vi "Frame Load Bmp and Img.vi"(8 "error in (no error)":errorcluster, 9 "PNG Path":path, 10 "File String":string, 11 "LF2R IDE in":refnum<class "Main Panel.lvclass">) -> (0 "error out":errorcluster, 3 "LF2R IDE out":refnum<class "Main Panel.lvclass">)   [LabVIEW 2018, in "Main Panel.lvlib" / "Main Panel.lvclass"]
uses:
  Main Panel.lvclass
  <vilib>/picture/picture.llb/imagedata.ctl
  Main Panel.lvclass/Main Panel.ctl
  Frame Analizer/Data Parser.lvclass
  Picture Process/Picture Process.lvclass
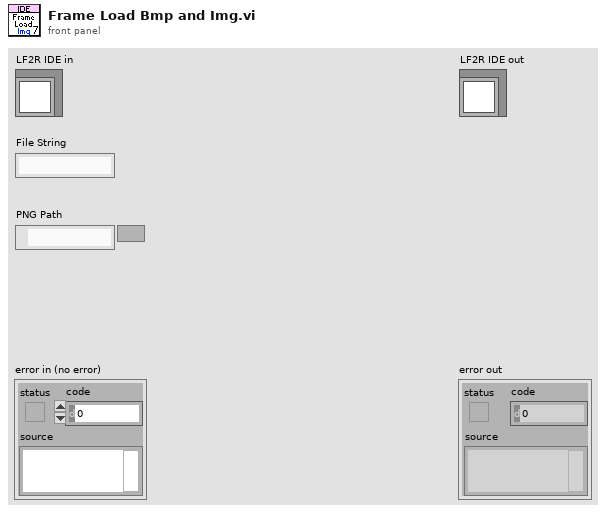
[diagram p1: front panel]
types:
  T1 = typedef "imagedata.ctl" = cluster{"image type":i32, "image depth":i32, "image":u8[], "mask":u8[], "colors":u32[], "Rectangle":cluster{"left":i16, "top":i16, "right":i16, "bottom":i16}}
  T2 = typedef "Data Parser.lvclass/Bmp data.ctl" = cluster{"File Data":T3[], "resized":string, "default_centerx":string, "default_centery":string}
  T3 = typedef "Data Parser.lvclass/Bmp File Data.ctl" = cluster{"Pic Start":i32, "Pic End":i32, "Json Path":string, "w":i32, "h":i32, "row":i32, "col":i32}
  T4 = typedef "Image Json Parser.lvclass/Img Json Data.ctl" = cluster{"frames":T5[], "meta":T6}
  T5 = typedef "Image Json Parser.lvclass/Img Json Frames.ctl" = cluster{"frame":cluster{"x":i32, "y":i32, "w":i32, "h":i32}, "rotated":bool, "trimmed":bool, "spriteSourceSize":cluster{"x":i32, "y":i32, "w":i32, "h":i32}, "sourceSize":cluster{"w":i32, "h":i32}}
  T6 = typedef "Image Json Parser.lvclass/Img Json Meta.ctl" = cluster{"app":string, "version":string, "image":string, "format":string, "size":cluster{"w":i32, "h":i32}, "scale":string}
  T7 = cluster{"image data":T1, "24-bit pixmap":u32[][]}
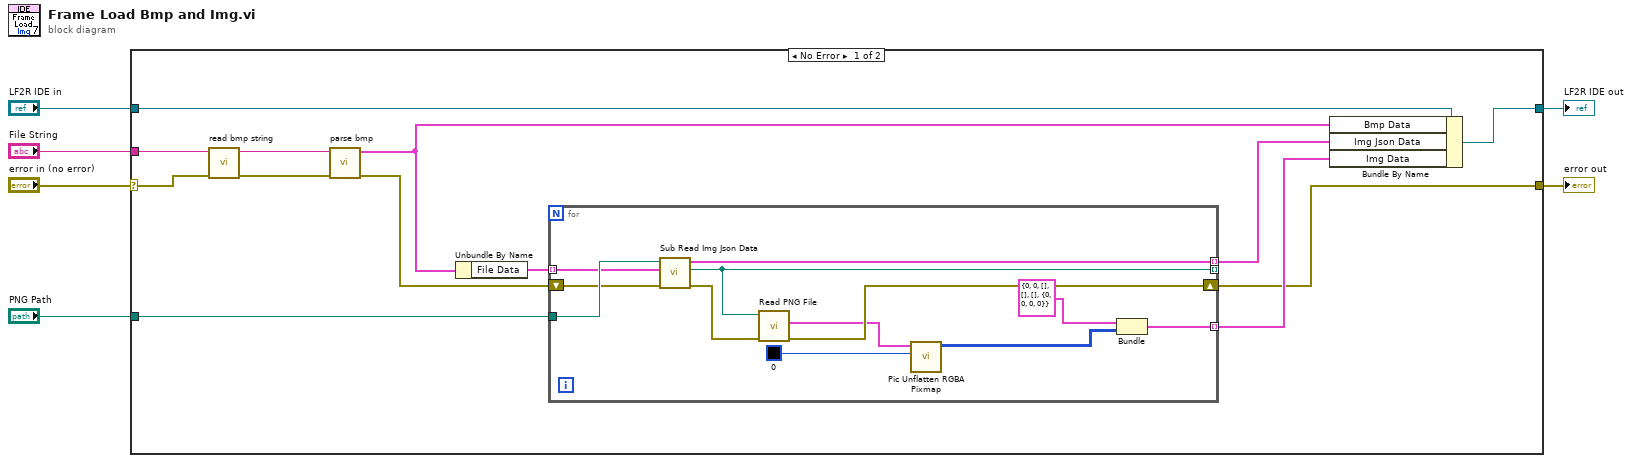
[diagram p0: block diagram]
diagram:
  n1 = case shown="No Error" "error in (no error)" {
    selector: "error in (no error)" -> [w15 w33]
    tunnel: [w7 w33] -> w5
    tunnel: [w14 w32] -> w3
    tunnel: "LF2R IDE in" -> [w19 w32]
    tunnel: "File String" -> [w16 _]
    tunnel: "PNG Path" -> [w13 _]
    frame No Error {
      n2 = call "read bmp string.vi"("error in"=w15, "file string"=w16) -> ("error out"=w17:errorcluster, "<bmp> string"=w18:string)  [unwired: 7 in, 1 out]
      n3 = call "parse bmp.vi"("error in (no error)"=w17, "<bmp> string"=w18) -> ("error out"=w9:errorcluster, "bmp data"=w12:T2)  [unwired: 8 in]
      n4 = Unbundle By Name(w12) -> ("File Data"=w11:T3[])
      n5 = for {
        tunnel: w13 -> [w31]
        tunnel: [w28] -> w10 mode=indexing
        shift-right: [w22] -> w7
        shift-left: w9 -> [w30]
        tunnel: w11 -> [w29] mode=indexing
        tunnel: [w27] -> _ mode=indexing
        tunnel: [w25] -> w8 mode=indexing
        n6 = call "Sub Read Img Json Data.vi"("error in"=w30, "File Data"=w29, "PNG Path"=w31) -> ("error out"=w26:errorcluster, "Image Path"=w27:path, "Json Data"=w28:T4)  [unwired: 6 in]
        n7 = call <vilib>:"Read PNG File.vi"("error in (no error)"=w26, "path to PNG file"=w27) -> ("error out"=w22:errorcluster, "image data"=w21:T1)  [unwired: 7 in, 1 out]
        n8 = call "Pic Unflatten RGBA Pixmap.vi"("BG Color"=u32 0, "32-bit image data (ARGB)"=w21) -> ("24-bit pixmap"=w24:u32[][])  [unwired: 8 in, 1 out]
        n9 = Bundle("image data"=T1 {"image type"=0, "image depth"=0, "image"=[], "mask"=[], "colors"=[], "Rectangle"={"left"=0, "top"=0, "right"=0, "bottom"=0}}, "24-bit pixmap"=w24) -> (w25:T7)  [unwired: 1 in]
      }
      n10 = Bundle By Name(cluster=w19, "Bmp Data"=w12, "Img Json Data"=w10, "Img Data"=w8) -> (w14:refnum<class "Main Panel.lvclass">)
    }
    frame Error {
    }
  }
  "error out" <- w5
  "LF2R IDE out" <- w3
